vi "CheckState.vi"(8 "error in (no error)":errorcluster, 11 "name":string) -> (0 "error out":errorcluster, 3 "active":bool)   [LabVIEW 2017, in "McsaResourceScheduler.lvlib"]
uses:
  <vilib>/addons/InsightCM/Devices/Shared/Mcsa/McsaResourceScheduler/McsaResourceScheduler.lvlib
  <vilib>/addons/InsightCM/Devices/Shared/Mcsa/McsaResourceScheduler/controls/InternalAction.ctl
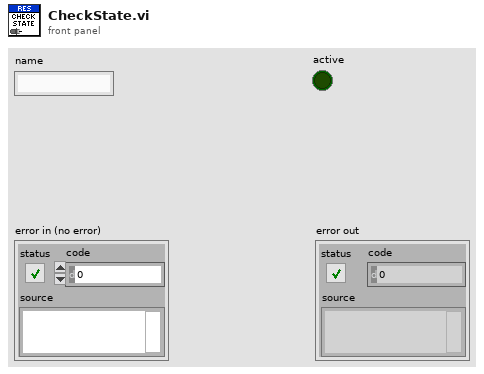
[diagram p1: front panel]
types:
  T1 = typedef "McsaResourceScheduler.lvlib/InternalAction.ctl" = enum16{"Initialize", "Register", "Unregister", "Get"}
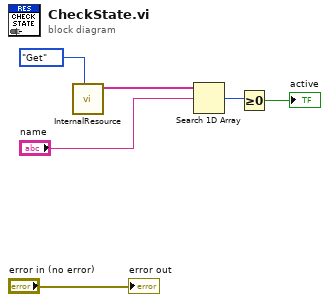
[diagram p0: block diagram]
diagram:
  n1 = call <vilib>:"InternalResource.vi"("action"=InternalAction."Get") -> ("active list"=w4:string[])  [unwired: 9 in, 1 out]
  n2 = Search 1D Array(1D array=w4, element="name") -> (index of element=w2:i32)  [unwired: 1 in]
  n3 = Greater Or Equal To 0?(x=w2) -> (x >= 0?=→"active":bool)
  "error out" <- "error in (no error)"
